vi "Log_Data.vi"(0 "File_Path_In":path, 5 "Input_Size (in kb)":i64, 11 "Error_In":errorcluster) -> (4 "File_Path_Out":path, 15 "Error_Out":errorcluster)   [LabVIEW 2021]
doc: "This VI logs the data that are generated to text file."
uses:
  Controls/Operation_Select_Queue.ctl
  <vilib>/regexp/Match Regular Expression.xnode
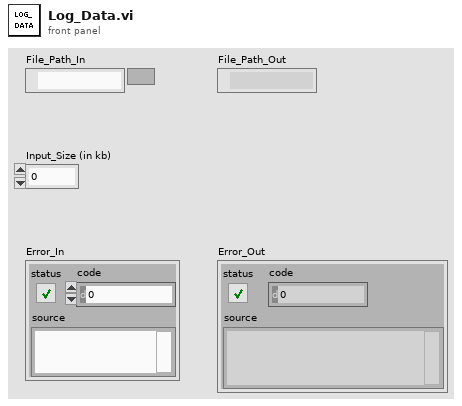
[diagram p1: front panel]
types:
  T1 = typedef "Operation_Select_Queue.ctl" = enum16{"Initialize", "Enqueue", "Dequeue", "Preview"}
  T2 = enum16{"open", "replace", "create", "open or create", "replace or create", "replace or create with confirmation"}
  T3 = typedef "Data.ctl" = cluster{"Generated_Data":dbl, "Time_Stamp":string}
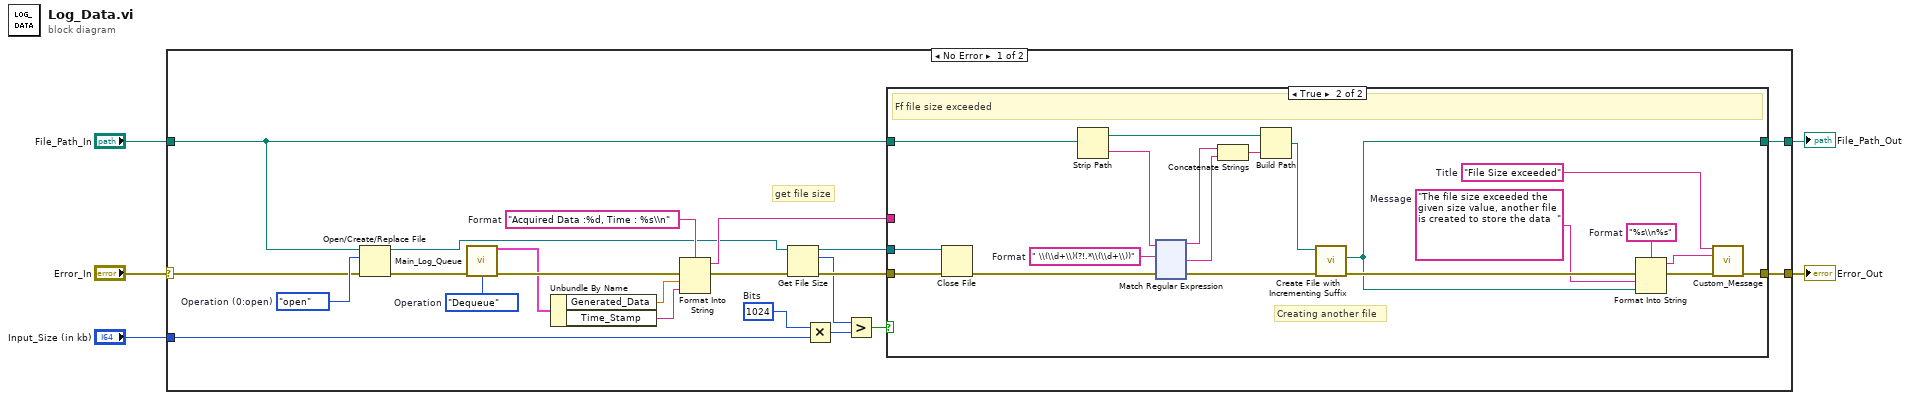
[diagram p0: block diagram]
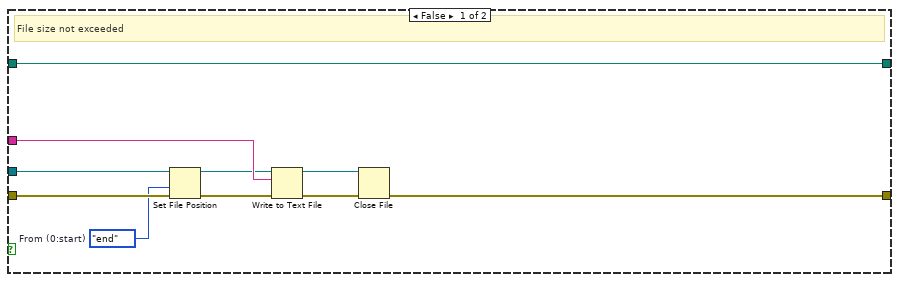
[diagram p2: hidden frame]
diagram:
  n1 = case shown="No Error" "Error_In" {
    selector: "Error_In" -> [w19 w176]
    tunnel: "File_Path_In" -> [w12 w175]
    tunnel: [w11 w176] -> w5
    tunnel: "Input_Size (in kb)" -> [w7 _]
    tunnel: [w10 w175] -> w2
    frame No Error {
      w6 = i64 1024  # Bits
      w20 = "Acquired Data :%d, Time : %s\\n"  # Format
      w25 = Operation_Select_Queue."Dequeue"  # Operation
      w27 = T2."open"  # Operation (0:open)
      # "get file size"
      n2 = Open/Create/Replace File(file path (use dialog)=w12, error in=w19, operation (0:open)=w27) -> (refnum out=w9:refnum<file>, error out=w26:errorcluster)  [unwired: 3 in, 1 out]
      n3 = call "Main_Log_Queue.vi"("Error_In"=w26, "Operation"=w25) -> ("Generated_Data_Out"=w23:T3, "Error_Out"=w24:errorcluster)  [unwired: 9 in, 3 out]
      n4 = Unbundle By Name(w23) -> ("Generated_Data"=w22:dbl, "Time_Stamp"=w21:string)
      n5 = Format Into String(format string=w20, error in=w24, w22, w21) -> (resulting string=w13:string, error out=w18:errorcluster)  [unwired: 1 in]
      n6 = Get File Size(file=w9, error in=w18) -> (refnum out=w16:refnum<file>, size (in bytes)=w14:i64, 0:w17:errorcluster)
      n7 = Multiply(x=w6, y=w7) -> (x*y=w8:i64)
      n8 = Greater?(x=w14, y=w8) -> (0:w15:bool)
      n9 = case shown="True" w15 {
        tunnel: [w35 w41] -> w11
        tunnel: w17 -> [w32 w57]
        tunnel: w16 -> [w31 w56]
        tunnel: w13 -> [w37 _]
        tunnel: w12 -> [w33 w55]
        tunnel: [w33 w39] -> w10
        frame False {
          w28 = enum16{"start", "end", "current"}."end"  # From (0:start)
          # "File size not exceeded"
          n10 = Set File Position(refnum=w31, from (0:start)=w28, error in=w32) -> (refnum out=w30:refnum<file>, error out=w29:errorcluster)  [unwired: 1 in]
          n11 = Write to Text File(file (use dialog)=w30, text=w37, error in=w29) -> (refnum out=w34:refnum<file>, error out=w36:errorcluster)  [unwired: 1 in, 1 out]
          n12 = Close File(refnum=w34, error in=w36) -> (error out=w35:errorcluster)  [unwired: 1 out]
        }
        frame True {
          w43 = "%s\\n%s"  # Format
          w45 = "File Size exceeded"  # Title
          w40 = "The file size exceeded the given size value, another file is created to store the data  "  # Message
          w51 = " \\(\\d+\\)(?!.*\\(\\d+\\))"  # Format
          # "Creating another file"
          # "Ff file size exceeded"
          n13 = Close File(refnum=w56, error in=w57) -> (error out=w46:errorcluster)  [unwired: 1 out]
          n14 = Strip Path(path=w55) -> (stripped path=w53:path, name=w52:string)
          n15 = xnode "Match Regular Expression"("input string"=w52, "regular expression"=w51, "error in"=w46) -> ("before match"=w50:string, "after match"=w49:string, "error out"=w47:errorcluster)  [unwired: 3 in, 2 out]
          n16 = Concatenate Strings(w50, w49) -> (w48:string)
          n17 = Build Path(base path=w53, name or relative path=w48) -> (appended path=w54:path)
          n18 = call <vilib>:"Create File with Incrementing Suffix.vi"("error in (no error)"=w47, "file path"=w54) -> ("error out"=w44:errorcluster, "actual path"=w39:path)  [unwired: 7 in, 1 out]
          n19 = Format Into String(format string=w43, error in=w44, w40, w39) -> (resulting string=w38:string, error out=w42:errorcluster)  [unwired: 1 in]
          n20 = call "Custom_Message.vi"("Title"=w45, "Message"=w38, "Error_In"=w42) -> ("Error_Out"=w41:errorcluster)  [unwired: 11 in, 1 out]
        }
      }
    }
    frame Error {
    }
  }
  "Error_Out" <- w5
  "File_Path_Out" <- w2
